vi "Triplet Cartesian Center Sort.vi"(1 "Triplet 2":T1, 2 "Triplet 1":T1) -> (0 "x < y?":bool)   [LabVIEW 2025]
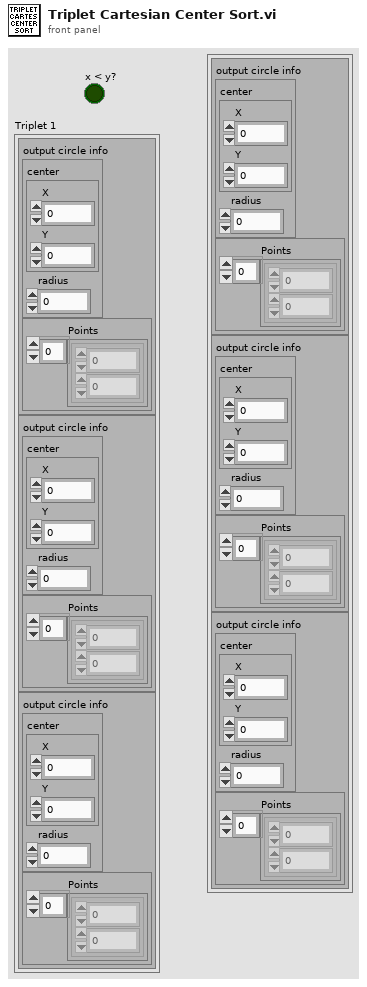
[diagram p1: front panel]
types:
  T1 = cluster{cluster{"output circle info":cluster{"center":cluster{"X":sgl, "Y":sgl}, "radius":sgl}, cluster{"Points":cluster{dbl, dbl}[]}}, cluster{"output circle info":cluster{"center":cluster{"X":sgl, "Y":sgl}, "radius":sgl}, cluster{"Points":cluster{dbl, dbl}[]}}, cluster{"output circle info":cluster{"center":cluster{"X":sgl, "Y":sgl}, "radius":sgl}, cluster{"Points":cluster{dbl, dbl}[]}}}
  T2 = cluster{"output circle info":cluster{"center":cluster{"X":sgl, "Y":sgl}, "radius":sgl}, cluster{"Points":cluster{dbl, dbl}[]}}
  T3 = cluster{"center":cluster{"X":sgl, "Y":sgl}, "radius":sgl}
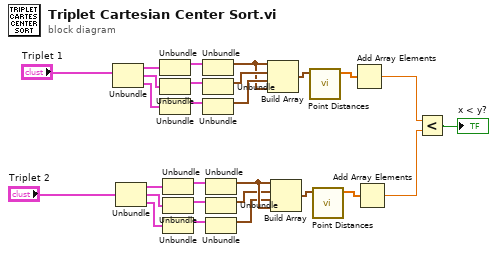
[diagram p0: block diagram]
diagram:
  n1 = Unbundle("Triplet 1") -> (w26:T2, w24:T2, w25:T2)
  n2 = Unbundle("Triplet 2") -> (w5:T2, w7:T2, w6:T2)
  n3 = Unbundle(w26) -> ("output circle info"=w23:T3)  [unwired: 1 out]
  n4 = Unbundle(w24) -> ("output circle info"=w22:T3)  [unwired: 1 out]
  n5 = Unbundle(w25) -> ("output circle info"=w21:T3)  [unwired: 1 out]
  n6 = Unbundle(w5) -> ("output circle info"=w8:T3)  [unwired: 1 out]
  n7 = Unbundle(w7) -> ("output circle info"=w9:T3)  [unwired: 1 out]
  n8 = Unbundle(w6) -> ("output circle info"=w10:T3)  [unwired: 1 out]
  n9 = Unbundle(w23) -> ("center"=w17:cluster{"X":sgl, "Y":sgl})  [unwired: 1 out]
  n10 = Unbundle(w22) -> ("center"=w19:cluster{"X":sgl, "Y":sgl})  [unwired: 1 out]
  n11 = Unbundle(w21) -> ("center"=w18:cluster{"X":sgl, "Y":sgl})  [unwired: 1 out]
  n12 = Unbundle(w8) -> ("center"=w14:cluster{"X":sgl, "Y":sgl})  [unwired: 1 out]
  n13 = Unbundle(w9) -> ("center"=w12:cluster{"X":sgl, "Y":sgl})  [unwired: 1 out]
  n14 = Unbundle(w10) -> ("center"=w13:cluster{"X":sgl, "Y":sgl})  [unwired: 1 out]
  n15 = Build Array(w17, w19, w18, w17) -> (w20:cluster{"X":sgl, "Y":sgl}[])
  n16 = Build Array(w14, w12, w13, w14) -> (w11:cluster{"X":sgl, "Y":sgl}[])
  n17 = call "Point Distances.vi"("Points"=w20) -> ("Distances"=w16:sgl[])  [unwired: 10 in]
  n18 = call "Point Distances.vi"("Points"=w11) -> ("Distances"=w15:sgl[])  [unwired: 10 in]
  n19 = Add Array Elements(numeric array=w16) -> (sum=w3:sgl)
  n20 = Add Array Elements(numeric array=w15) -> (sum=w2:sgl)
  n21 = Less?(x=w3, y=w2) -> (x < y?=→"x < y?":bool)
